vi "Welcome.vi"() -> ()   [LabVIEW 2017]
doc: "Use this template to build a producer/consumer design pattern with events to produce queue items. Use this design pattern instead of the User Interface Event Handler pattern for user interfaces when you want to execute code asynchronously in response to an event without slowing the user interface responsiveness."
panel:
  in  "Enqueue Element":bool
  # "提供优质可靠的测控技术服务"
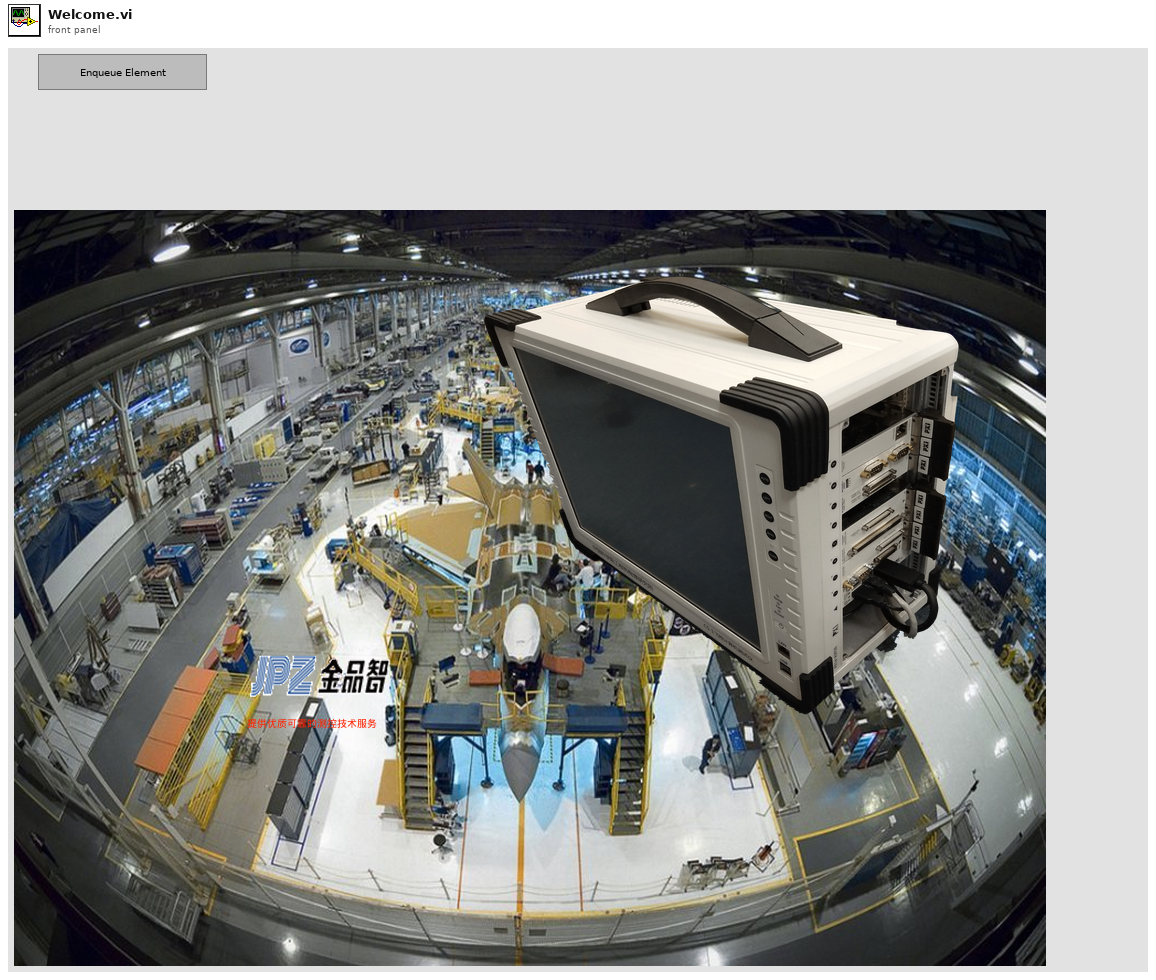
[diagram p1: front panel]
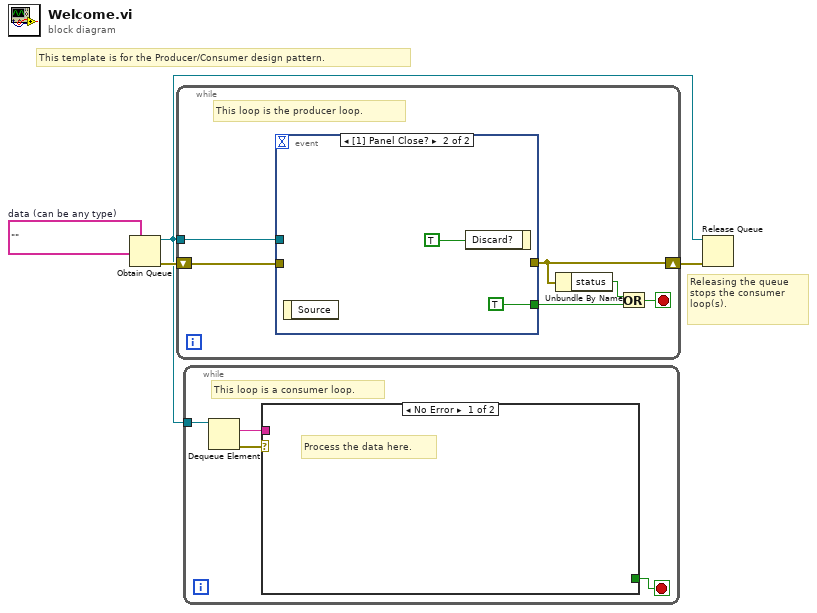
[diagram p0: block diagram]
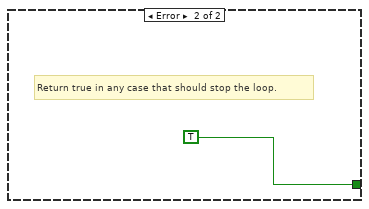
[diagram p2: hidden frame]
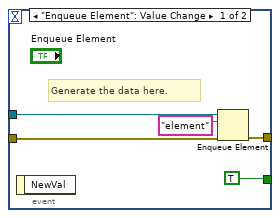
[diagram p3: hidden frame]
diagram:
  w2 = ""  # data (can be any type)
  # "Releasing the queue stops the consumer loop(s)."
  # "This template is for the Producer/Consumer design pattern."
  n1 = Obtain Queue(element data type=w2) -> (queue out=w1:refnum<queue>, error out=w4:errorcluster)  [unwired: 4 in, 1 out]
  n2 = while {
    shift-right: [w6] -> w3
    shift-left: w4 -> [w9]
    tunnel: w1 -> [w10]
    stop <- w7 stop-if-true
    # "This loop is the producer loop."
    n3 = event shown="[1] Panel Close?" {
      selector: _ -> [_ _]
      dyn-events: _ -> [_ _]
      timeout: _ -> [_ _]
      tunnel: w10 -> [w15 _]
      tunnel: w9 -> [w14 _]
      tunnel: [w13 _] -> w6
      tunnel: [TRUE TRUE] -> w8
      event "Enqueue Element": Value Change {
        # "Generate the data here."
        n4 = event-data() -> ()  [unwired: 1 in, 1 out]
        n5 = Enqueue Element(queue=w15, element="element", error in (no error)=w14) -> (error out=w13:errorcluster)  [unwired: 1 in, 2 out]
      }
      event Panel Close? {
        n6 = event-data() -> ()  [unwired: 1 in, 1 out]
        n7 = event-data("Discard?"=TRUE) -> ()  [unwired: 1 in, 1 out]
      }
    }
    n8 = Unbundle By Name(w6) -> ("status"=w5:bool)
    n9 = Or(x=w5, y=w8) -> (x .or. y?=w7:bool)
  }
  n10 = while {
    tunnel: w1 -> [w21]
    stop <- w18 stop-if-true
    # "This loop is a consumer loop."
    n11 = Dequeue Element(queue=w21) -> (element=w19:string, error out=w20:errorcluster)  [unwired: 2 in, 2 out]
    n12 = case shown="No Error" w20 {
      tunnel: w19 -> [_ _]
      tunnel: [_ TRUE] -> w18
      frame No Error {
        # "Process the data here."
      }
      frame Error {
        # "Return true in any case that should stop the loop."
      }
    }
  }
  n13 = Release Queue(queue=w1, error in (no error)=w3) -> ()  [unwired: 1 in, 3 out]
